vi "Create Project FIFOs - Top.vi"(7 "Current Bus Number":i32, 8 "error in (no error)":errorcluster, 9 "Device Channels":i32[](array[numeric]), 10 "LabVIEW Project to Script":path) -> (0 "error out":errorcluster)   [LabVIEW 2014, in "SPI Engine Scripting.lvlib"]
doc: "Creates a single \"FIFOs\" project folder and two project FIFOs for each channel on the bus."
uses:
  SPI Engine Scripting.lvlib
  State Machine/Controls/Values for Naming.ctl
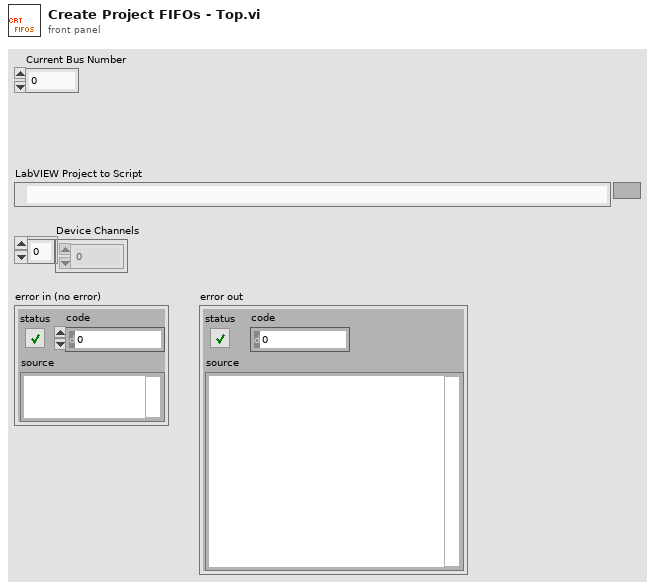
[diagram p1: front panel]
types:
  T1 = typedef "SPI Engine Scripting.lvlib/Values for Naming.ctl" = cluster{"Bus Number":i32, "Device Number":i32, "Channel Number":i32}
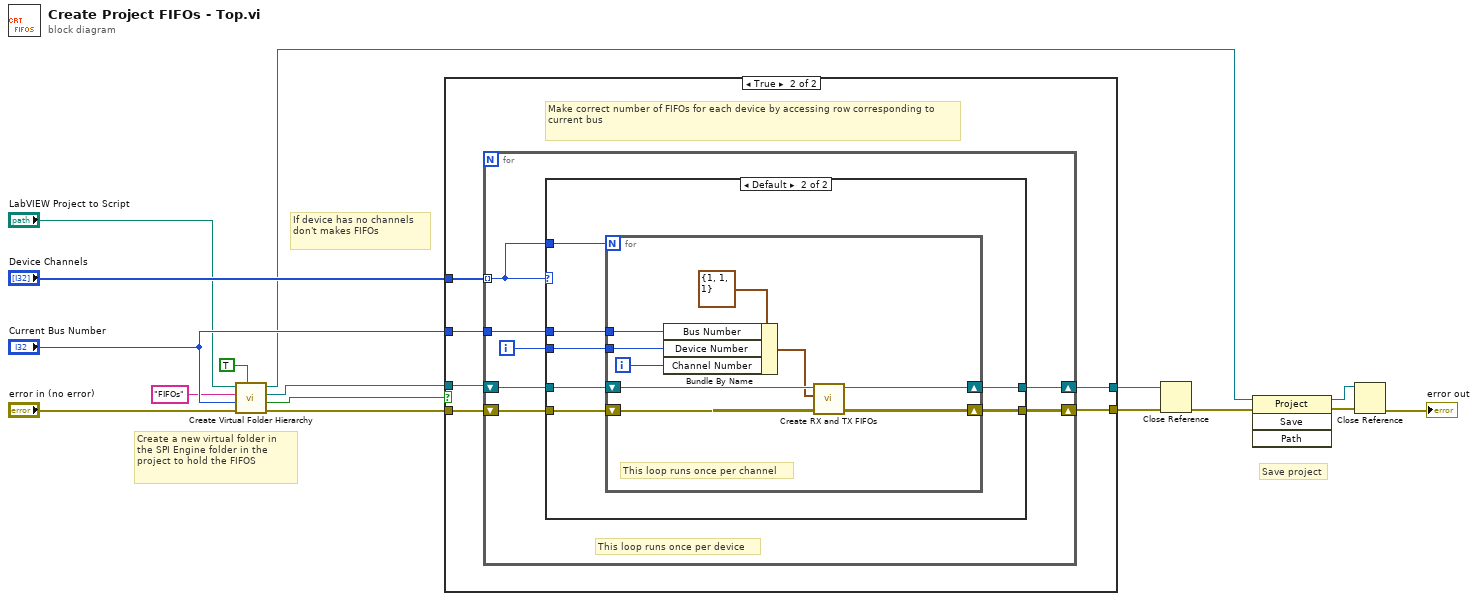
[diagram p0: block diagram]
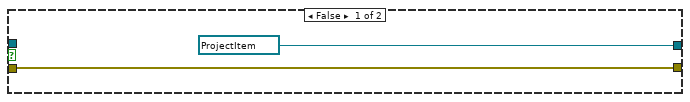
[diagram p2: hidden frame]
diagram:
  # "If device has no channels don't makes FIFOs"
  # "Save project"
  # "Create a new virtual folder in the SPI Engine folder in the project to hold the FIFOS"
  n1 = call "Create Virtual Folder Hierarchy.vi"("Create Sub-Bus Folder (F)"=TRUE, "error in"="error in (no error)", "Bus Number"="Current Bus Number", "Virtual Folder Name"="FIFOs", "Path to Project"="LabVIEW Project to Script") -> ("error out"=w11:errorcluster, "FPGA Target Found"=w13:bool, "New Virtual Folder"=w14:refnum<vi>, "Project:Open"=w10:refnum<vi>)  [unwired: 3 in]
  n2 = case shown="True" w13 {
    tunnel: [w18 w24] -> w9
    tunnel: w11 -> [w18 w23]
    tunnel: [refnum<vi> refnum ("Comm FIFOs Virtual Folder") w22] -> w12
    tunnel: w14 -> [_ w21]
    tunnel: "Device Channels" -> [_ w19]
    tunnel: "Current Bus Number" -> [_ w20]
    frame False {
    }
    frame True {
      # "Make correct number of FIFOs for each device by accessing row corresponding to current bus"
      n3 = for {
        shift-right: [w31] -> w24
        shift-left: w23 -> [w30]
        tunnel: w19 -> [w25] mode=indexing
        shift-right: [w29] -> w22
        shift-left: w21 -> [w28]
        tunnel: w20 -> [w26]
        i -> [w27]
        # "This loop runs once per device"
        n4 = case shown="Default" w25 {
          tunnel: [w33 w40] -> w31
          tunnel: w30 -> [w33 w39]
          tunnel: [w32 w38] -> w29
          tunnel: w28 -> [w32 w37]
          tunnel: w27 -> [_ w36]
          tunnel: w25 -> [_ w35]
          tunnel: w26 -> [_ w34]
          frame 0 {
          }
          frame Default {
            n5 = for {
              N: w35 -> [_]
              shift-right: [w49] -> w40
              shift-left: w39 -> [w48]
              shift-right: [w47] -> w38
              shift-left: w37 -> [w46]
              tunnel: w36 -> [w43]
              tunnel: w34 -> [w42]
              i -> [w44]
              # "This loop runs once per channel"
              n6 = Bundle By Name(cluster=T1 {"Bus Number"=1, "Device Number"=1, "Channel Number"=1} ("Values for Naming"), "Bus Number"=w42, "Device Number"=w43, "Channel Number"=w44) -> (w41:T1)
              n7 = call "Create RX and TX FIFOs.vi"("error in"=w48, "Values for Naming"=w41, "New Virtual Folder"=w46) -> ("error out"=w49:errorcluster, "Comm FIFOs Virtual Folder"=w47:refnum<vi>)  [unwired: 7 in]
            }
          }
        }
      }
    }
  }
  n8 = Close Reference(reference=w12, error in (no error)=w9) -> (error out=w5:errorcluster)
  n9 = invoke class="Project" method="Save"(reference=w10, error in=w5) -> (reference out=w7:refnum<vi>, error out=w6:errorcluster)  [unwired: 2 in, 2 out]
  n10 = Close Reference(reference=w7, error in (no error)=w6) -> (error out=→"error out":errorcluster)
